vi "insert and update save variable.vi"(8 "error in":errorcluster, 10 "device name":string, 11 "checkbox value":i32) -> (0 "error out":errorcluster)   [LabVIEW 2020]
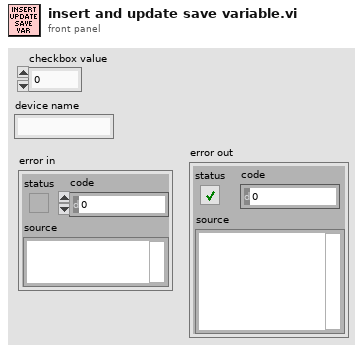
[diagram p1: front panel]
types:
  T1 = typedef "mysql_authentication.ctl" = cluster{"User":string, "Password":string, "Database":string}
  T2 = cluster{"Port":u16, "IP Address":string, "Authentication":T1}
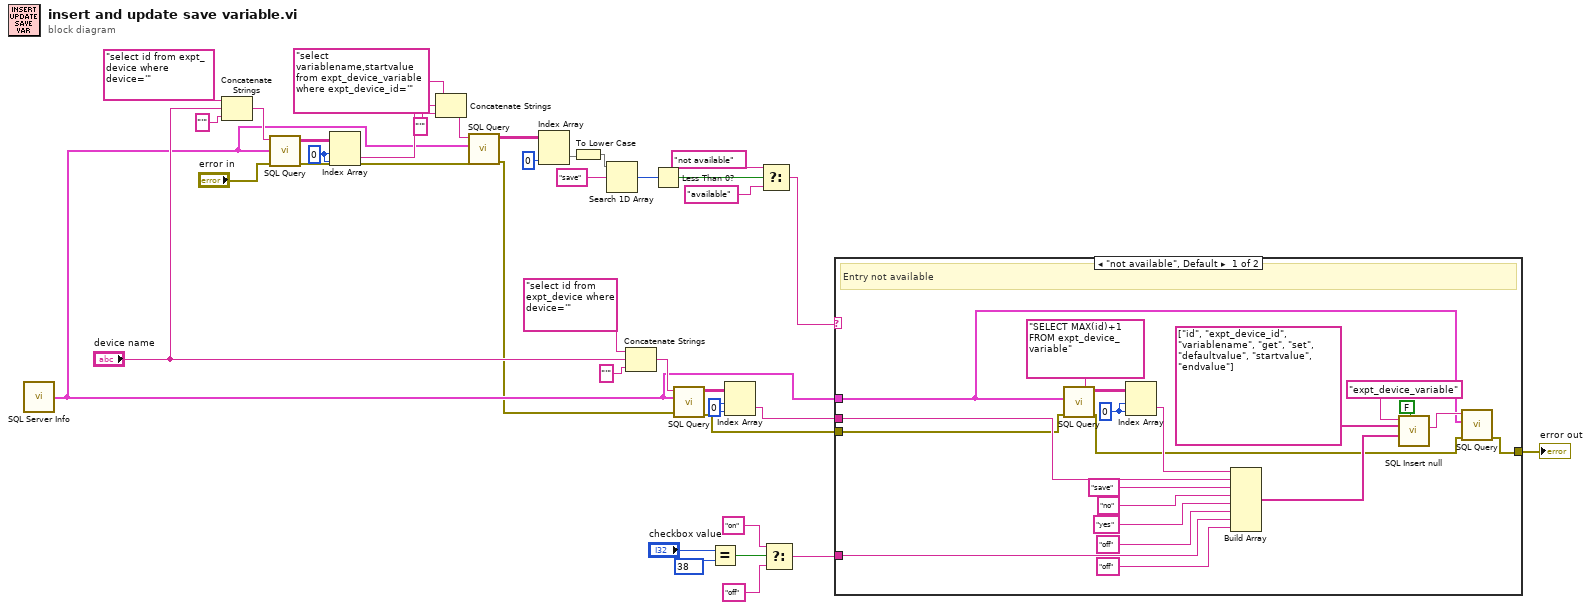
[diagram p0: block diagram]
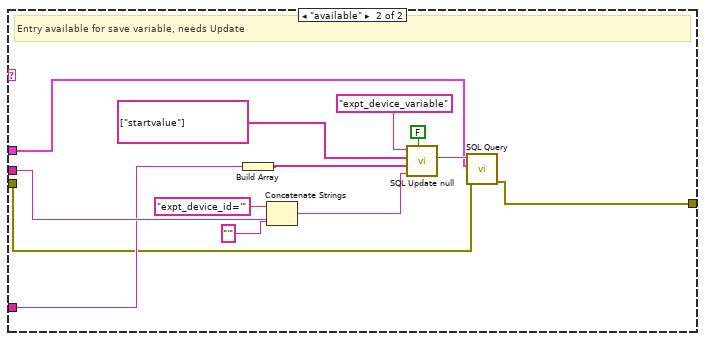
[diagram p2: hidden frame]
diagram:
  w21 = 0 ("index (row)")
  w32 = 0
  n1 = call "SQL Server Info.vi"() -> ("SQL Server Info"=w4:T2)
  n2 = Concatenate Strings("select id from expt_device where device='" ("Query"), "device name", "'" ("Query")) -> (w22:string)
  n3 = call "SQL Query.vi"("error in (no error)"="error in", "SQL Server Info"=w4, "Query"=w22) -> ("error out"=w19:errorcluster, "data"=w20:string[][])  [unwired: 7 in]
  n4 = Index Array(array=w20, index (row)=w21, index (col)=w21) -> (element=w13:string)
  n5 = Concatenate Strings("select variablename,startvalue from expt_device_variable where expt_device_id='" ("Query"), w13, "'" ("Query")) -> (w11:string)
  n6 = call "SQL Query.vi"("error in (no error)"=w19, "SQL Server Info"=w4, "Query"=w11) -> ("error out"=w2:errorcluster, "data"=w10:string[][])  [unwired: 7 in]
  n7 = Index Array(array=w10, index (col)=0 ("disabled index (col)")) -> (element=w17:string[])  [unwired: 1 in]
  n8 = To Lower Case(string=w17) -> (all lower case string=w18:string[])
  n9 = Search 1D Array(1D array=w18, element="save") -> (index of element=w9:i32)  [unwired: 1 in]
  n10 = Concatenate Strings("select id from expt_device where device='" ("Query"), "device name", "'" ("Query")) -> (w30:string)
  n11 = Less Than 0?(x=w9) -> (x < 0?=w8:bool)
  n12 = call "SQL Query.vi"("error in (no error)"=w2, "SQL Server Info"=w4, "Query"=w30) -> ("error out"=w26:errorcluster, "data"=w31:string[][])  [unwired: 7 in]
  n13 = Equal?(x="checkbox value", y=38) -> (x = y?=w36:bool)
  n14 = Index Array(array=w31, index (row)=w32, index (col)=w32) -> (element=w27:string)
  n15 = Select(t="not available" ("element"), s=w8, f="available" ("element")) -> (s? t:f=w1:string)
  n16 = Select(t="on" ("available entry?"), s=w36, f="off" ("available entry?")) -> (s? t:f=w33:string)
  n17 = case shown="\"not available\", Default" w1 {
    tunnel: w33 -> [w48 w63]
    tunnel: w4 -> [w41 w65]
    tunnel: w27 -> [w45 w67]
    tunnel: w26 -> [w44 w61]
    tunnel: [w39 w60] -> w25
    frame "not available", Default {
      w57 = 0 ("disabled index (col)")
      # "Entry not available"
      n18 = call "SQL Query.vi"("error in (no error)"=w44, "SQL Server Info"=w41, "Query"="SELECT MAX(id)+1 FROM expt_device_variable") -> ("error out"=w40:errorcluster, "data"=w56:string[][])  [unwired: 7 in]
      n19 = Index Array(array=w56, index (row)=w57, index (col)=w57) -> (element=w53:string)
      n20 = Build Array(w53, w45, "save" ("element"), "no" ("element"), "yes" ("element"), "off" ("element"), w48, "off" ("element")) -> (w46:string[])
      n21 = call "SQL Insert null.vi"("Use Empty String As Ignore? (T)"=FALSE, "Values"=w46, "Column Names"=string[] ["id", "expt_device_id", "variablename", "get", "set", "defaultvalue", "startvalue", "endvalue"], "Table"="expt_device_variable") -> ("Query String"=w42:string)  [unwired: 7 in]
      n22 = call "SQL Query.vi"("error in (no error)"=w40, "SQL Server Info"=w41, "Query"=w42) -> ("error out"=w39:errorcluster)  [unwired: 7 in, 1 out]
    }
    frame "available" {
      # "Entry available for save variable, needs Update"
      n23 = Build Array(w63) -> (w62:string[])
      n24 = Concatenate Strings("expt_device_id='" ("Where clause"), w67, "'" ("Query")) -> (w66:string)
      n25 = call "SQL Update null.vi"("Use Empty String as Ignore? (T)"=FALSE, "Where clause"=w66, "Values"=w62, "Column Names"=string[] ["startvalue"], "Table"="expt_device_variable") -> ("Query String"=w69:string)  [unwired: 6 in]
      n26 = call "SQL Query.vi"("error in (no error)"=w61, "SQL Server Info"=w65, "Query"=w69) -> ("error out"=w60:errorcluster)  [unwired: 7 in, 1 out]
    }
  }
  "error out" <- w25
